vi "CLD 2  Elapsed Time Express Caller Exercise.vi"() -> ()   [LabVIEW 2014]
doc: "CLD-Übung 2"
panel:
  out "Zeit ist verstrichen":bool
  out "Verstrichene Zeit (s)":dbl format="%#.2g"
  out "Fehler (Ausgang)":errorcluster
  in  "Zielzeit (s)":dbl=4.0
  in  "Autom. zurücksetzen (F)":bool=TRUE
  in  "Fehler (Eingang, kein Fehler)":errorcluster
  in  "Timer-Modus":T1(ring)
  in  "Stopp":bool
  # "Aufrufer der FGV"
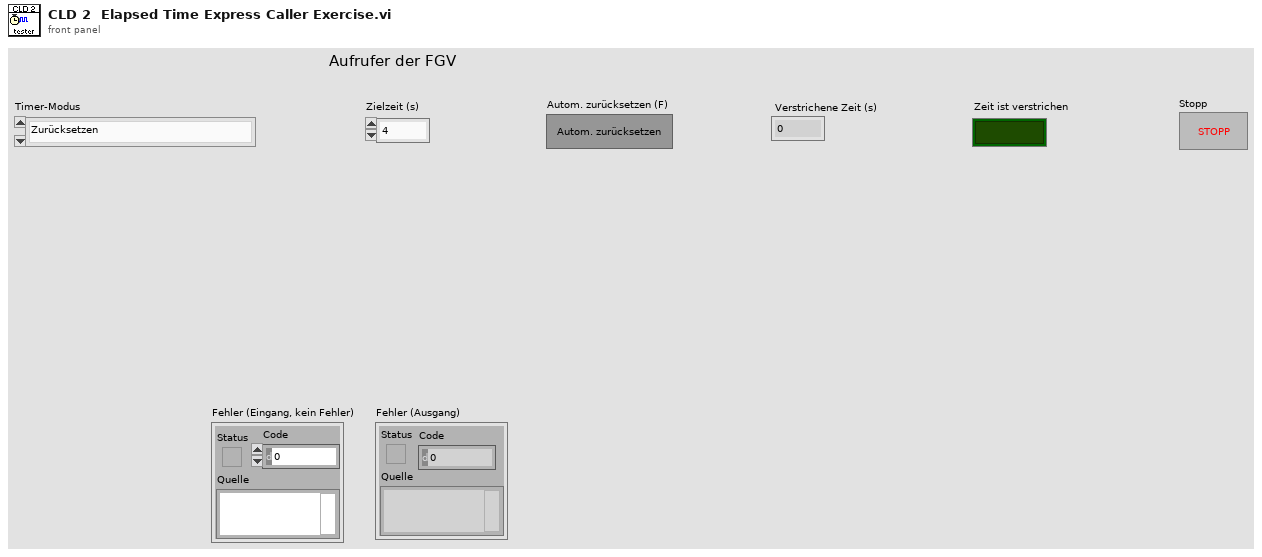
[diagram p1: front panel]
types:
  T1 = enum16{"Zurücksetzen", "Status abfragen", "Autom. Zurücksetzen festlegen"}
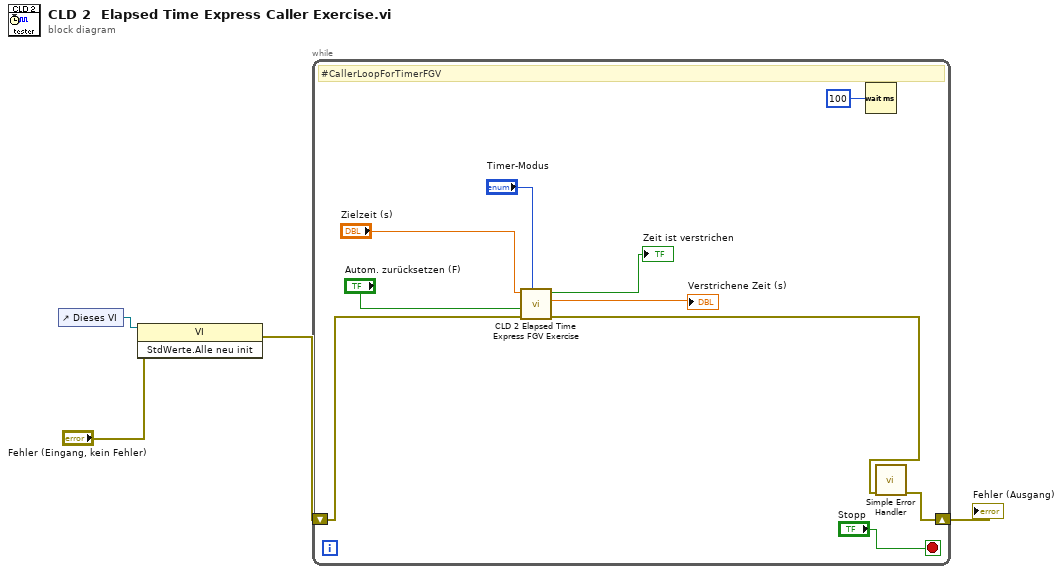
[diagram p0: block diagram]
diagram:
  n1 = control-ref of="Dieses VI"() -> (w3:refnum<vi>)
  n2 = invoke class="VI" method="StdWerte.Alle neu init"(reference=w3, error in="Fehler (Eingang, kein Fehler)") -> (error out=w1:errorcluster)  [unwired: 1 in, 2 out]
  n3 = while {
    shift-right: [w13] -> w4
    shift-left: w1 -> [w12]
    stop <- "Stopp" stop-if-true
    # "#CallerLoopForTimerFGV"
    n4 = call "CLD 2 Elapsed Time Express FGV Exercise.vi"("Timer-Modus"="Timer-Modus", "Fehler (Eingang, kein Fehler)"=w12, "Autom. zurücksetzen (F)"="Autom. zurücksetzen (F)", "Zielzeit (s)"="Zielzeit (s)") -> ("Fehler (Ausgang)"=w11:errorcluster, "Verstrichene Zeit (s)"=→"Verstrichene Zeit (s)":dbl, "Zeit ist verstrichen"=→"Zeit ist verstrichen":bool)  [unwired: 5 in]
    n5 = Wait (ms)(milliseconds to wait=u32 100 ("Zu wartende ms")) -> ()  [unwired: 1 out]
    n6 = call <vilib>:"Simple Error Handler.vi"("error in (no error)"=w11) -> ("error out"=w13:errorcluster)  [unwired: 4 in, 4 out]
  }
  "Fehler (Ausgang)" <- w4
